vi "60Percent.vi"(0 "In":dbl) -> (7 "Out":dbl)   [LabVIEW 2019]
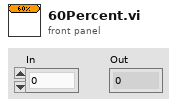
[diagram p1: front panel]
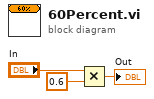
[diagram p0: block diagram]
diagram:
  n1 = Multiply(x="In", y=0.6) -> (x*y=→"Out":dbl)
